vi "Stitching Test.vi"() -> ()   [LabVIEW 2017, in "Processing.lvlib"]
uses:
  Processing.lvlib
  File IO/Controls/Params.ctl
  File IO/File IO.lvlib
panel:
  out "error out":errorcluster
  in  "input cluster":T2
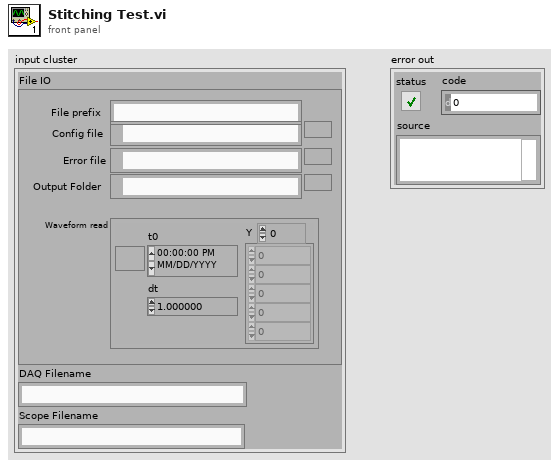
[diagram p1: front panel]
types:
  T1 = typedef "File IO.lvlib/Params.ctl" = cluster{"Output Folder":path, "Error file":path, "Config file":path, "File prefix":string, "Waveform read":waveform(dbl)}
  T2 = cluster{"File IO":T1, "DAQ Filename":string, "Scope Filename":string}
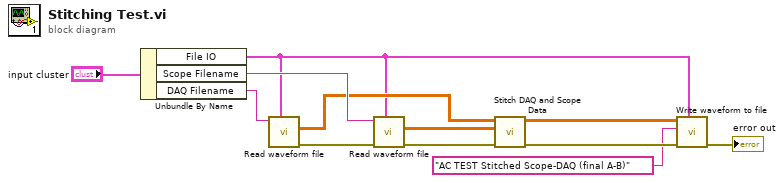
[diagram p0: block diagram]
diagram:
  n1 = Unbundle By Name("input cluster") -> ("File IO"=w2:T1, "Scope Filename"=w10:string, "DAQ Filename"=w11:string)
  n2 = call "Read waveform file.vi"("File IO parameters"=w2, "Dataset name"=w11) -> ("error out"=w12:errorcluster, "all rows"=w8:dbl[][])  [unwired: 7 in, 1 out]
  n3 = call "Read waveform file.vi"("File IO parameters"=w2, "error in"=w12, "Dataset name"=w10) -> ("error out"=w9:errorcluster, "all rows"=w7:dbl[][])  [unwired: 6 in, 1 out]
  n4 = call "Stitch DAQ and Scope Data.vi"("error in (no error)"=w9, "Scope Ch1 (final A-B)"=w7, "DAQ DOD (final)"=w8) -> ("error out"=w4:errorcluster, "data & time array"=w5:dbl[][])  [unwired: 7 in]
  n5 = call "Write waveform to file.vi"("File IO parameters"=w2, "error in"=w4, "Dataset name"="AC TEST Stitched Scope-DAQ (final A-B)", "Data"=w5) -> ("error out"=→"error out":errorcluster)  [unwired: 7 in]
